vi "GET_FIFO.vi"(0 "TCP Network Connection in":refnum<k5>, 2 "N":u32=100, 5 "error in (no error)":errorcluster) -> (14 "TCP Network Connection out":refnum<k5>, 16 "Oscilloscope":u32[](graph), 18 "Status":u8[](array[numeric]), 19 "error out":errorcluster)   [LabVIEW 2019]
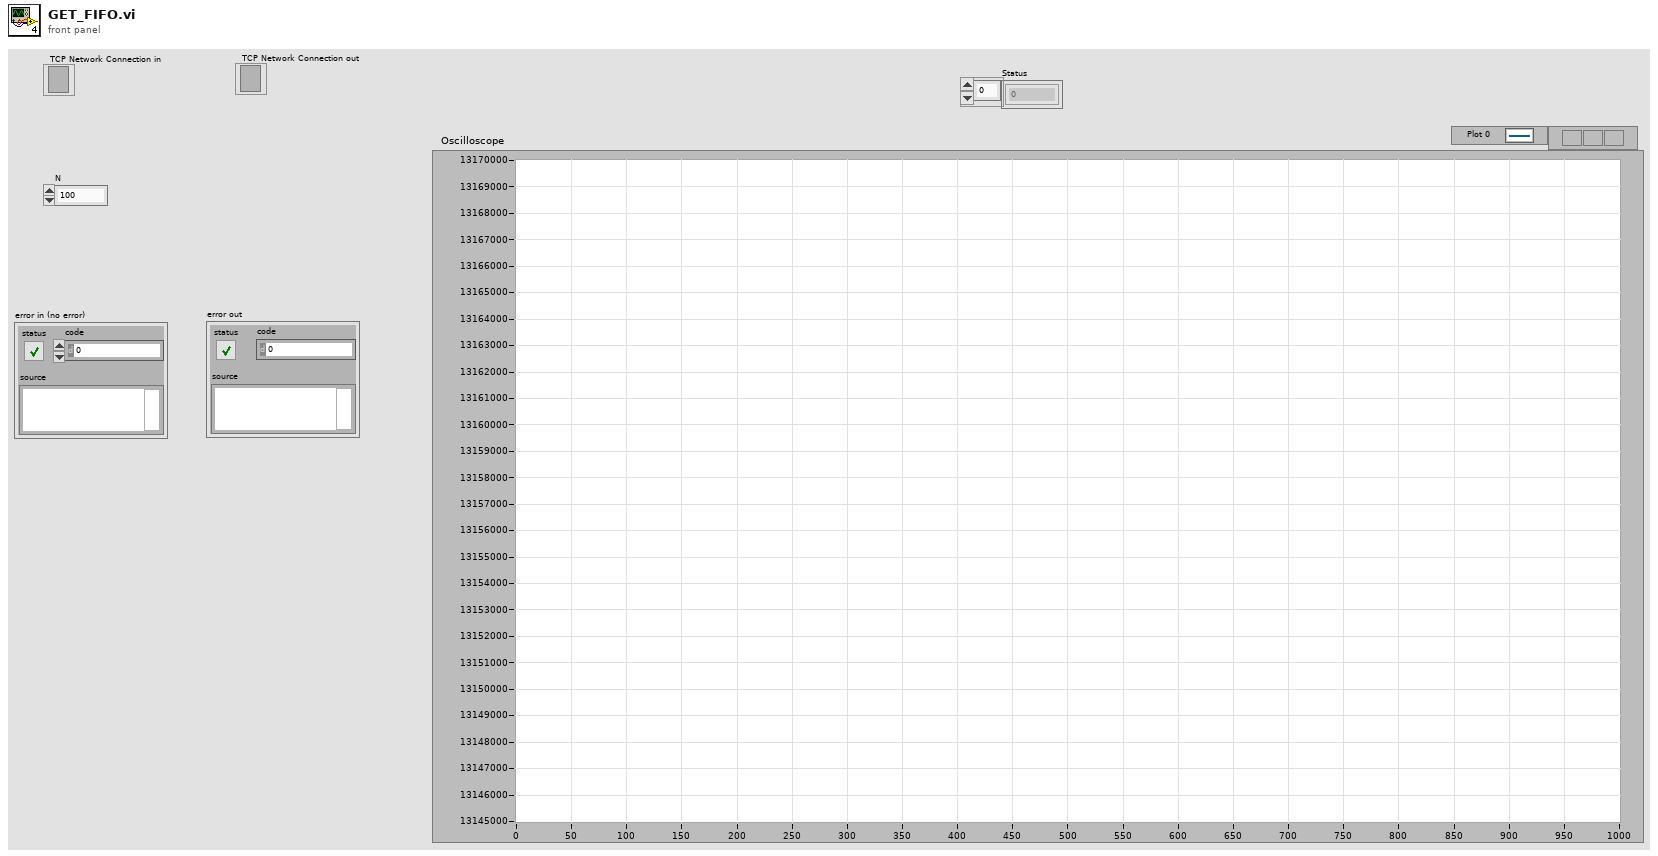
[diagram p1: front panel]
types:
  T1 = enum16{"big-endian, network order", "native, host order", "little-endian"}
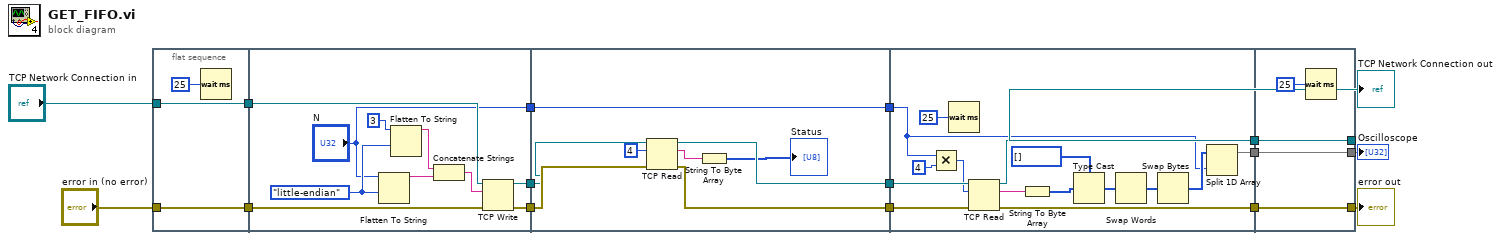
[diagram p0: block diagram]
diagram:
  n1 = flat-sequence {
    tunnel: [w18] -> w12
    tunnel: [w19] -> w11
    tunnel: "error in (no error)" -> [w19]
    tunnel: "TCP Network Connection in" -> [w18]
    tunnel: w12 -> [w29]
    tunnel: w11 -> [w28]
    tunnel: [w27] -> w6
    tunnel: [w26] -> w5
    tunnel: ["N"] -> w3
    tunnel: w6 -> [w33]
    tunnel: w5 -> [w36]
    tunnel: [w35] -> w4
    tunnel: w3 -> [w37]
    tunnel: [w37] -> w2
    tunnel: [w34] -> w1
    tunnel: w4 -> [w51]
    tunnel: w2 -> [w39]
    tunnel: [w50] -> w9
    tunnel: [w49] -> w8
    tunnel: [w40] -> w7
    tunnel: w1 -> [w52]
    tunnel: [w54] -> w10
    tunnel: [w55] -> w14
    tunnel: [w56] -> w13
    tunnel: w9 -> [w56]
    tunnel: w8 -> [w55]
    tunnel: w7 -> [w54]
    frame #0 {
      n2 = Wait (ms)(milliseconds to wait=u32 25) -> ()  [unwired: 1 out]
    }
    frame #1 {
      w24 = T1."little-endian" ("byte order (0:big-endian, network order)")
      n3 = Flatten To String(anything="N", byte order (0:big-endian, network order)=w24) -> (data string=w25:string)  [unwired: 2 in, 2 out]
      n4 = Flatten To String(anything=u32 3 ("element"), byte order (0:big-endian, network order)=w24) -> (data string=w22:string)  [unwired: 2 in, 2 out]
      n5 = Concatenate Strings(w22, w25) -> (w21:string)
      n6 = TCP Write(connection ID=w29, data in=w21, error in (no error)=w28) -> (connection ID out=w27:refnum<k5>, error out=w26:errorcluster)  [unwired: 1 in, 1 out]
    }
    frame #2 {
      n7 = TCP Read(connection ID=w33, bytes to read=4, error in (no error)=w36) -> (connection ID out=w34:refnum<k5>, data out=w32:string, error out=w35:errorcluster)  [unwired: 2 in]
      n8 = String To Byte Array(string=w32) -> (unsigned byte array=→"Status":u8[])
    }
    frame #3 {
      n9 = Multiply(x=w39, y=u32 4) -> (x*y=w47:u32)
      n10 = Wait (ms)(milliseconds to wait=u32 25) -> ()  [unwired: 1 out]
      n11 = TCP Read(connection ID=w52, bytes to read=w47, error in (no error)=w51) -> (connection ID out=w50:refnum<k5>, data out=w38:string, error out=w49:errorcluster)  [unwired: 2 in]
      n12 = String To Byte Array(string=w38) -> (unsigned byte array=w45:u8[])
      n13 = Type Cast(type=u32[] [], x=w45) -> (*(type *) &x=w43:u32[])
      n14 = Swap Words(1:w43) -> (0:w42:u32[])
      n15 = Swap Bytes(anything=w42) -> (byte swapped=w41:u32[])
      n16 = Split 1D Array(array=w41, index=w39) -> (first subarray=w40:u32[])  [unwired: 1 out]
    }
    frame #4 {
      n17 = Wait (ms)(milliseconds to wait=u32 25) -> ()  [unwired: 1 out]
    }
  }
  "error out" <- w14
  "TCP Network Connection out" <- w13
  "Oscilloscope" <- w10
